vi "PID Lead-Lag (DBL).vi"(4 "reinitialize? (F)":bool, 5 "time unit":u16(ring)=1 items=["second", "minute"], 6 "dt (s)":dbl=-1.0 format="%.3f", 7 "output range":cluster{"output high":dbl, "output low":dbl}={"output high"=100.0, "output low"=-100.0} {"output low" format="%.2f"; "output high" format="%.2f"}, 8 "tuning parameters":T1={"gain"=1.0, "lag time"=0.01, "lead time"=0.0} {"lead time" format="%.3f"; "lag time" format="%.3f"; "gain" format="%.3f"}, 9 "input":dbl format="%.2f") -> (0 "dt out (s)":dbl format="%.3f", 3 "output":dbl format="%.2f")   [LabVIEW 2020, in "NI_PID_pid.lvlib"]
doc: "Implements a PID controller with a lead/lag function, which is generally used as a dynamic compensator in feedforward control schemes. This VI uses a positional algorithm and is an approximation of a true exponential lead/lag. Use the DBL instance of this VI to implement a single control loop. Use the DBL Array instance to implement parallel multi-loop control."
uses:
  <vilib>/addons/control/pid/NI_PID_pid.lvlib
panel:
  # "where:\nTlead: lead time\nTlag: lag time\nK: gain\nU(s): input\nY(s): output"
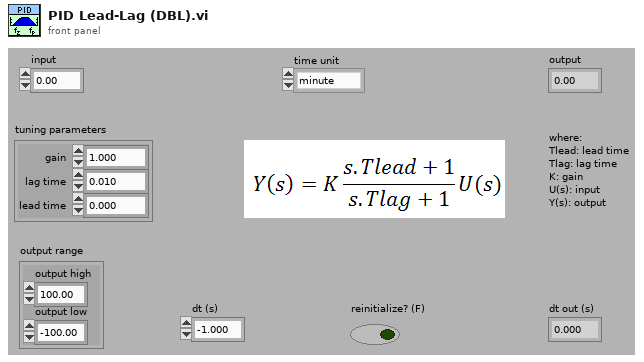
[diagram p1: front panel]
types:
  T1 = cluster{"gain":dbl, "lag time":dbl, "lead time":dbl}
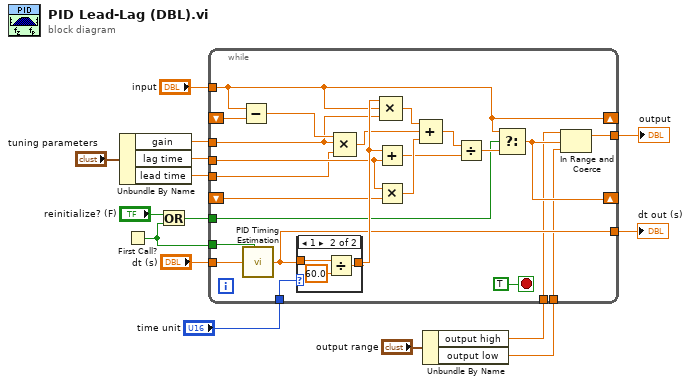
[diagram p0: block diagram]
diagram:
  n1 = Unbundle By Name("tuning parameters") -> ("gain"=w9:dbl, "lag time"=w8:dbl, "lead time"=w7:dbl)
  n2 = First Call?() -> (First Call?: T/F=w12:bool)
  n3 = Or(x="reinitialize? (F)", y=w12) -> (x .or. y?=w14:bool)
  n4 = Unbundle By Name("output range") -> ("output high"=w2:dbl, "output low"=w1:dbl)
  n5 = while {
    tunnel: w14 -> [w30]
    shift-left: _ -> [w36]
    shift-right: [w29] -> _
    shift-left: _ -> [w38]
    shift-right: [w19] -> _
    tunnel: "dt (s)" -> [w26]
    tunnel: w12 -> [w25]
    tunnel: [w24] -> w11
    tunnel: [w23] -> w10
    tunnel: w9 -> [w22]
    tunnel: w8 -> [w21]
    tunnel: w7 -> [w20]
    tunnel: "input" -> [w19]
    tunnel: "time unit" -> [w18]
    tunnel: w2 -> [w17]
    tunnel: w1 -> [w16]
    stop <- TRUE stop-if-true
    n6 = Subtract(x=w19, y=w38) -> (x-y=w37:dbl)
    n7 = call <vilib>:"PID Timing Estimation.vi"("Initialize?"=w25, "dt (s) in"=w26) -> ("dt (s) out"=w24:dbl)  [unwired: 7 in]
    n8 = case shown="1" w18 {
      tunnel: [w40 w42] -> w39
      tunnel: w24 -> [w40 w41]
      frame 0, Default {
      }
      frame 1 {
        n9 = Divide(x=w41, y=60.0) -> (x/y=w42:dbl)
      }
    }
    n10 = Compound Arithmetic op=MULTIPLY(w37, w22, w20) -> (w27:dbl)
    n11 = Add(x=w39, y=w21) -> (x+y=w32:dbl)
    n12 = Multiply(x=w21, y=w36) -> (x*y=w34:dbl)
    n13 = Compound Arithmetic op=MULTIPLY(w39, w19, w22) -> (w35:dbl)
    n14 = Compound Arithmetic op=ADD(w35, w27, w34) -> (w33:dbl)
    n15 = Divide(x=w33, y=w32) -> (x/y=w31:dbl)
    n16 = Select(t=w19, s=w30, f=w31) -> (s? t:f=w29:dbl)
    n17 = In Range and Coerce(upper limit=w17, x=w29, lower limit=w16) -> (coerced(x)=w23:dbl)  [unwired: 1 out]
  }
  "dt out (s)" <- w11
  "output" <- w10
